vi "Defence Cross.vi"() -> ()   [LabVIEW 2015]
uses:
  CrossDefenceStates.ctl
  Support/Global Objects.vi
panel:
  in  "DeclineTimeDecline":i32
  in  "FlatTimeFlat":i32
  in  "Motor Power":dbl=0.23
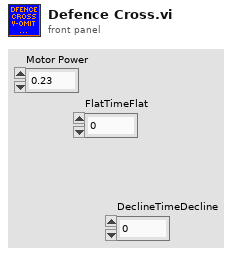
[diagram p1: front panel]
types:
  T1 = typedef "CrossDefenceStates.ctl" = enum16{"Driving Forward", "Wait for Decline", "Wait for Flat", "Stop"}
  T2 = typedef "NaxX Info.ctl" = cluster{"navX Device":T3, "Current Yaw":dbl, "Active":bool, "Current Roll":dbl}
  T3 = typedef "navX Library v2.lvlib/Z900_navX_DeviceTypeDef.ctl" = cluster{"Interface":cluster{"Protocol":T4, "Update Rate (4Hz-60Hz)":u8, "navX Open TypeDef":variant}, "Notify Packet":refnum<notifier>, "Loop VI Refnum":refnum<vi>, "Ready to Close Occurrence Refnum":refnum<k4>}
  T4 = typedef "navX Library v2.lvlib/Z900_navX_ProtocolTypeDef.ctl" = enum16{"SERIAL", "I2C", "SPI"}
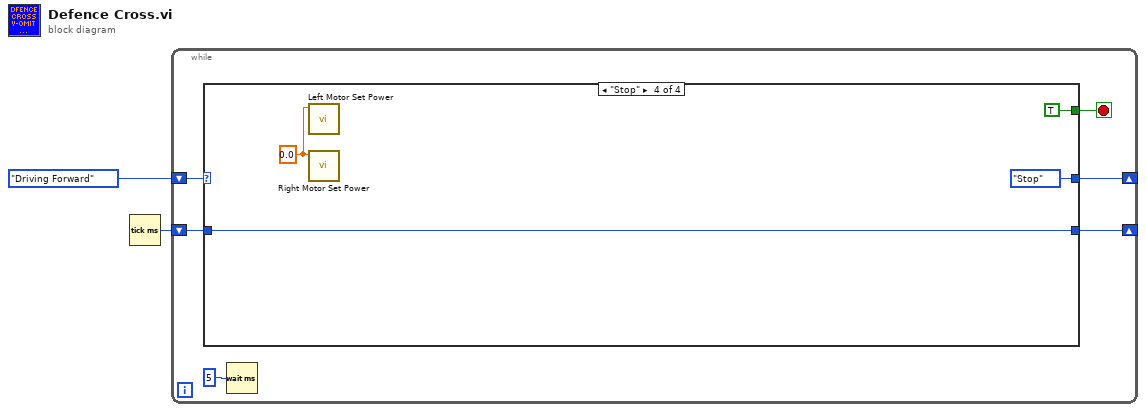
[diagram p0: block diagram]
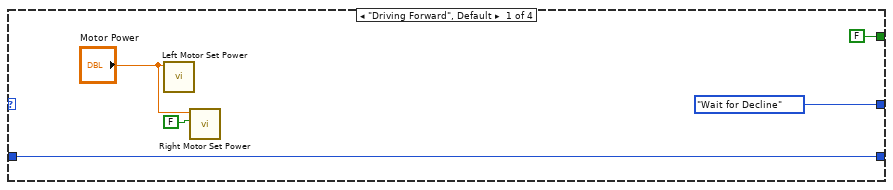
[diagram p2: hidden frame]
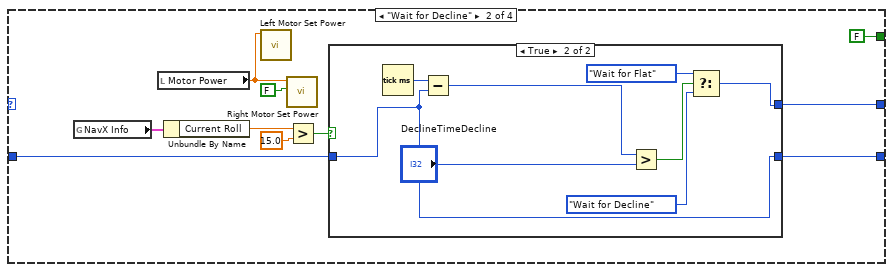
[diagram p3: hidden frame]
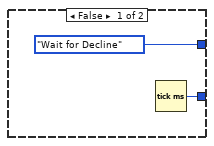
[diagram p4: hidden frame]
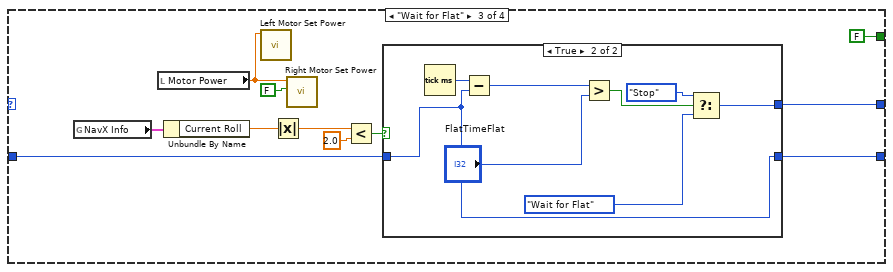
[diagram p5: hidden frame]
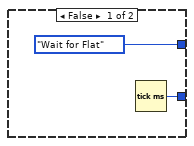
[diagram p6: hidden frame]
diagram:
  n1 = Tick Count (ms)() -> (millisecond timer value=w1:u32)
  n2 = while {
    shift-right: [w7] -> _
    shift-left: CrossDefenceStates."Driving Forward" -> [w8]
    shift-right: [w4] -> _
    shift-left: w1 -> [w3]
    stop <- w6 stop-if-true
    n3 = case shown="\"Stop\"" w8 {
      tunnel: [CrossDefenceStates."Wait for Decline" w14 w34 CrossDefenceStates."Stop"] -> w7
      tunnel: [FALSE FALSE FALSE TRUE] -> w6
      tunnel: [w9 w19 w36 w55] -> w4
      tunnel: w3 -> [w9 w20 w35 w55]
      frame "Driving Forward", Default {
        n4 = call "Left Motor Set Power.vi"("Output"="Motor Power") -> ()  [unwired: 10 in, 1 out]
        n5 = call "Right Motor Set Power.vi"("Disable Ramp"=FALSE, "Output"="Motor Power") -> ()  [unwired: 9 in, 1 out]
      }
      frame "Wait for Decline" {
        n6 = global read "Global Objects.vi" "NavX Info"() -> (w16:T2)
        n7 = local read "Motor Power"() -> (w21:dbl)
        n8 = Unbundle By Name(w16) -> ("Current Roll"=w17:dbl)
        n9 = call "Left Motor Set Power.vi"("Output"=w21) -> ()  [unwired: 10 in, 1 out]
        n10 = call "Right Motor Set Power.vi"("Disable Ramp"=FALSE, "Output"=w21) -> ()  [unwired: 9 in, 1 out]
        n11 = Greater?(x=w17, y=15.0) -> (0:w15:bool)
        n12 = case shown="True" w15 {
          tunnel: [w25 w26] -> w19
          tunnel: [CrossDefenceStates."Wait for Decline" w28] -> w14
          tunnel: w20 -> [_ w26]
          frame False {
            n13 = Tick Count (ms)() -> (millisecond timer value=w25:u32)
          }
          frame True {
            n14 = Tick Count (ms)() -> (millisecond timer value=w33:u32)
            n15 = Subtract(x=w33, y=w26) -> (x-y=w32:u32)
            n16 = Greater?(x=w32, y="DeclineTimeDecline") -> (0:w31:bool)
            n17 = Select(t=CrossDefenceStates."Wait for Flat", s=w31, f=CrossDefenceStates."Wait for Decline") -> (s? t:f=w28:T1)
          }
        }
      }
      frame "Wait for Flat" {
        n18 = global read "Global Objects.vi" "NavX Info"() -> (w43:T2)
        n19 = local read "Motor Power"() -> (w38:dbl)
        n20 = Unbundle By Name(w43) -> ("Current Roll"=w42:dbl)
        n21 = call "Left Motor Set Power.vi"("Output"=w38) -> ()  [unwired: 10 in, 1 out]
        n22 = Absolute Value(x=w42) -> (abs(x)=w41:dbl)
        n23 = call "Right Motor Set Power.vi"("Disable Ramp"=FALSE, "Output"=w38) -> ()  [unwired: 9 in, 1 out]
        n24 = Less?(x=w41, y=2.0) -> (x < y?=w37:bool)
        n25 = case shown="True" w37 {
          tunnel: [w46 w48] -> w36
          tunnel: w35 -> [_ w48]
          tunnel: [CrossDefenceStates."Wait for Flat" w49] -> w34
          frame False {
            n26 = Tick Count (ms)() -> (millisecond timer value=w46:u32)
          }
          frame True {
            n27 = Tick Count (ms)() -> (millisecond timer value=w54:u32)
            n28 = Subtract(x=w54, y=w48) -> (x-y=w53:u32)
            n29 = Greater?(x=w53, y="FlatTimeFlat") -> (0:w52:bool)
            n30 = Select(t=CrossDefenceStates."Stop", s=w52, f=CrossDefenceStates."Wait for Flat") -> (s? t:f=w49:T1)
          }
        }
      }
      frame "Stop" {
        w57 = 0.0 ("Output")
        n31 = call "Left Motor Set Power.vi"("Output"=w57) -> ()  [unwired: 10 in, 1 out]
        n32 = call "Right Motor Set Power.vi"("Output"=w57) -> ()  [unwired: 10 in, 1 out]
      }
    }
    n33 = Wait (ms)(milliseconds to wait=u32 5) -> ()  [unwired: 1 out]
  }
